vi "timeUnit.get.vi"(8 "error in (no error)":errorcluster, 11 "ts.epochOfTimeUnit in":refnum<class "ts.epochOfTimeUnit.lvclass">) -> (0 "error out":errorcluster, 2 "timeUnit":T1(ring), 3 "ts.epochOfTimeUnit out":refnum<class "ts.epochOfTimeUnit.lvclass">)   [LabVIEW 2020, in "ts.epochOfTimeUnit.lvclass"]
uses:
  ts.epochOfTimeUnit.lvclass
  ts.epochOfTimeUnit.lvclass/ts.epochOfTimeUnit.ctl
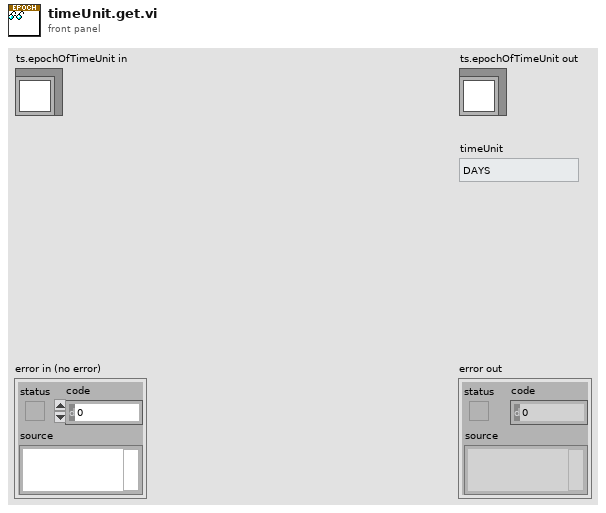
[diagram p1: front panel]
types:
  T1 = enum16{"DAYS", "HOURS", "MINUTES", "SECONDS", "MILLISECONDS", "MICROSECONDS", "NANOSECONDS", "PICOSECONDS"}
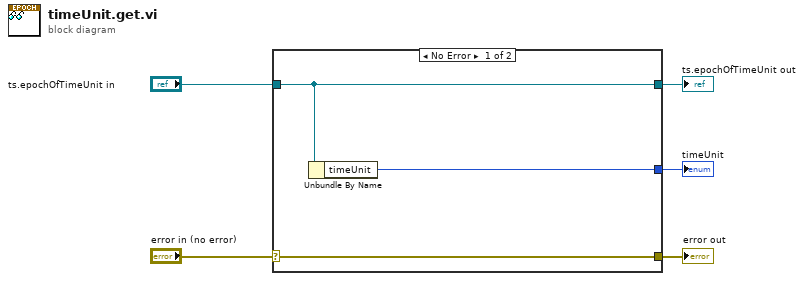
[diagram p0: block diagram]
diagram:
  n1 = case shown="No Error" "error in (no error)" {
    selector: "error in (no error)" -> [w8 w9]
    tunnel: [w8 w9] -> w4
    tunnel: [w7 w10] -> w2
    tunnel: "ts.epochOfTimeUnit in" -> [w7 w10]
    tunnel: [w6 _] -> w1
    frame No Error {
      n2 = Unbundle By Name(w7) -> ("timeUnit"=w6:T1)
    }
    frame Error {
    }
  }
  "error out" <- w4
  "ts.epochOfTimeUnit out" <- w2
  "timeUnit" <- w1
